vi "Error_5103.vi"(9 "Status":i32, 10 "Current Pos":i32, 11 "Target Pos":i32) -> (0 "error out":errorcluster)   [LabVIEW 2015, in "Tool Module.lvlib"]
uses:
  Tool Module.lvlib
  <vilib>/Utility/error.llb/Error Cluster From Error Code.vi
  <vilib>/ErrorRing/Error Ring.xnode
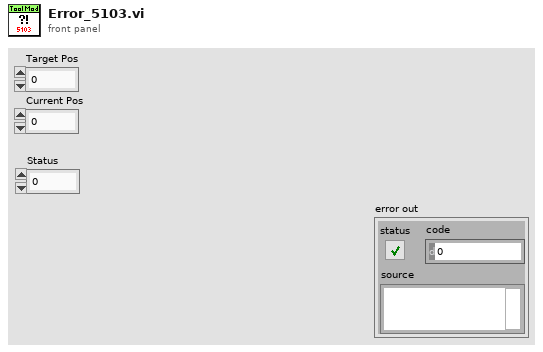
[diagram p1: front panel]
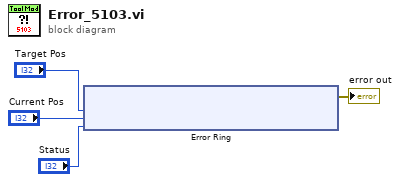
[diagram p0: block diagram]
diagram:
  n1 = xnode "Error Ring"("parameter 0"="Target Pos", "parameter 1"="Current Pos", "parameter 2"="Status") -> ("error out"=→"error out":errorcluster)
